vi "Set Process ID.vi"(10 "Process ID":string, 11 "CD_Process in":refnum<class "Process.lvclass">) -> (3 "CD_Process out":refnum<class "Process.lvclass">)   [LabVIEW 2019, in "TelemetryAsync Engine.lvlib" / "Process.lvclass"]
uses:
  Process.lvclass
  Process.lvclass/Process.ctl
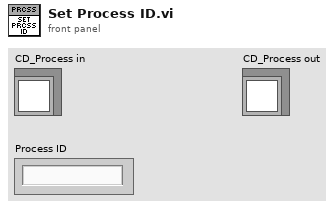
[diagram p1: front panel]
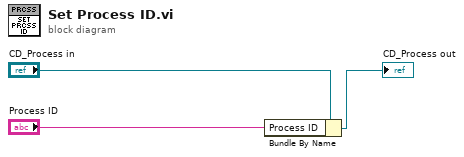
[diagram p0: block diagram]
diagram:
  n1 = Bundle By Name(cluster="CD_Process in", "Process ID"="Process ID") -> (→"CD_Process out":refnum<class "Process.lvclass">)
